vi "sensor cmd dock status.vi"(10 "status":string, 11 "device_handle":u32) -> (1 "function return":i32, 2 "status out":string, 3 "device_handle out":u32)   [LabVIEW 2019, in "apdm.lvlib"]
doc: "APDM_EXPORT int apdm_sensor_cmd_dock_status(apdm_device_handle_t device_handle, uint8_t *status);"
uses:
  apdm.lvlib
  Lee Lab/CP FES Walking 2018/Code/Working/LabVIEW/apdm.dll
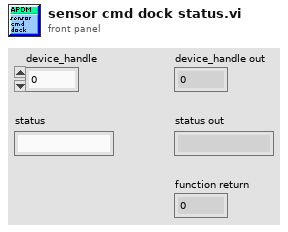
[diagram p1: front panel]
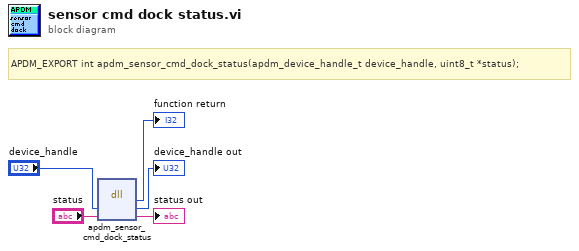
[diagram p0: block diagram]
diagram:
  # "APDM_EXPORT int apdm_sensor_cmd_dock_status(apdm_device_handle_t device_handle, uint8_t *status);"
  n1 = dll-call lib="C:/Users/jfalesi/Dropbox/Lee Lab/CP FES Walking 2018/Code/Working/LabVIEW/apdm.*" fn="apdm_sensor_cmd_dock_status"("device_handle"="device_handle", "status"="status") -> (→"function return":i32, "device_handle"=→"device_handle out":u32, "status"=→"status out":string)  [unwired: 3 in, 2 out]
